vi "Write Categories Order.vi"(8 "error in (no error)":errorcluster, 10 "Categories Order":T1(ring), 11 "Configuration in":refnum<class "Configuration.lvclass">) -> (0 "error out":errorcluster, 3 "Configuration out":refnum<class "Configuration.lvclass">)   [LabVIEW 2016, in "Configuration.lvlib" / "Configuration.lvclass"]
uses:
  <userlib>/Configuration Dialog Actor/Configuration.lvclass
  <userlib>/Configuration Dialog Actor/Configuration.lvclass/Configuration.ctl
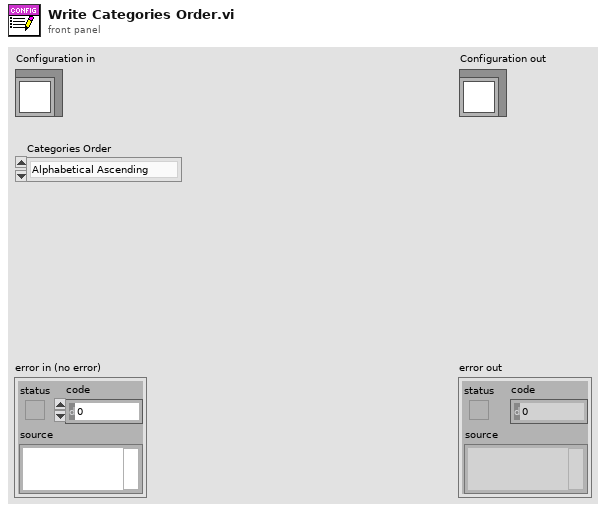
[diagram p1: front panel]
types:
  T1 = enum16{"Alphabetical Ascending", "Alphabetical Descending", "Chronological", "Reverse Chronological"}
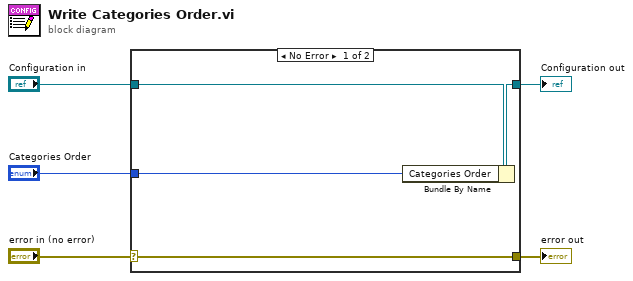
[diagram p0: block diagram]
diagram:
  n1 = case shown="No Error" "error in (no error)" {
    selector: "error in (no error)" -> [w9 w10]
    tunnel: [w9 w10] -> w4
    tunnel: [w7 w11] -> w2
    tunnel: "Configuration in" -> [w8 w11]
    tunnel: "Categories Order" -> [w6 _]
    frame No Error {
      n2 = Bundle By Name(cluster=w8, "Categories Order"=w6) -> (w7:refnum<class "Configuration.lvclass">)
    }
    frame Error {
    }
  }
  "error out" <- w4
  "Configuration out" <- w2
